vi "moving average.vi"(8 "error in (no error)":errorcluster, 10 "window size (3)":u32=3, 11 "x":dbl[](array[numeric])) -> (0 "error out":errorcluster, 3 "x smoothed":dbl[](array[numeric]))   [LabVIEW 2021]
uses:
  <vilib>/Analysis/2dsp.llb/1D Convolution (DBL).vi
  <vilib>/Analysis/NI_AALPro.lvlib
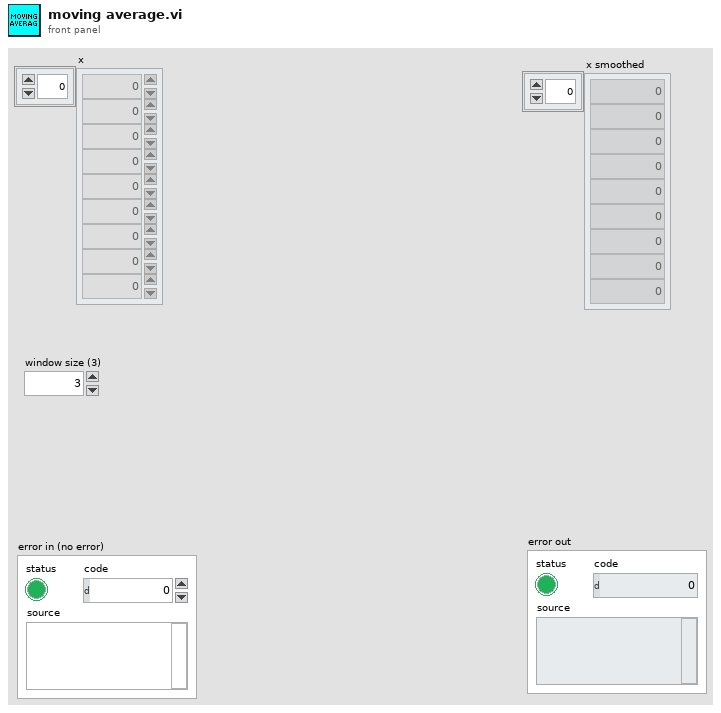
[diagram p1: front panel]
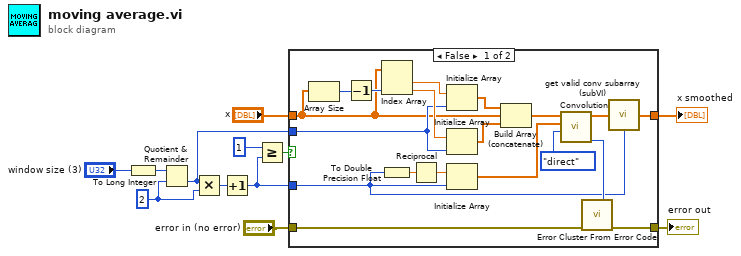
[diagram p0: block diagram]
diagram:
  w12 = 2 ("y")
  n1 = To Long Integer(number="window size (3)") -> (32bit integer=w10:i32)
  n2 = Quotient & Remainder(x=w10, y=w12) -> (floor(x/y)=w3:i32)  [unwired: 1 out]
  n3 = Multiply(x=w3, y=w12) -> (x*y=w2:i32)
  n4 = Increment(x=w2) -> (x+1=w8:i32)
  n5 = Greater Or Equal?(x=1, y=w8) -> (x >= y?=w7:bool)
  n6 = case shown="False" w7 {
    tunnel: w8 -> [w15 _]
    tunnel: [w14 w33] -> w5
    tunnel: "x" -> [w13 w33]
    tunnel: "error in (no error)" -> [w20 w32]
    tunnel: [w19 w32] -> w1
    tunnel: w3 -> [w16 _]
    frame False {
      n7 = Array Size(array=w13) -> (size(s)=w17:i32)
      n8 = Decrement(x=w17) -> (x-1=w28:i32)
      n9 = Index Array(array=w13, index #2=w28) -> (element #1=w29:dbl, element #2=w27:dbl)  [unwired: 1 in]
      n10 = To Double Precision Float(number=w15) -> (double precision float=w31:dbl)
      n11 = Reciprocal(x=w31) -> (1/x=w30:dbl)
      n12 = Initialize Array(w29, w16) -> (w26:dbl[])
      n13 = Initialize Array(w27, w16) -> (w25:dbl[])
      n14 = Initialize Array(w30, w15) -> (w24:dbl[])
      n15 = Build Array (concatenate)(w26, w13, w25) -> (w23:dbl[])
      n16 = call-poly <vilib>:"Convolution.vi"("algorithm"=enum32{"direct", "frequency domain"}."direct", "Y"=w24, "X"=w23) -> ("error"=w21:i32, "X * Y"=w18:dbl[])  [unwired: 7 in]
      n17 = call <vilib>:"Error Cluster From Error Code.vi"("error in (no error)"=w20, "error code (0)"=w21) -> ("error out"=w19:errorcluster)  [unwired: 7 in]
      n18 = call "get valid conv subarray (subVI).vi"("k size"=w15, "X * k"=w18) -> ("X * k valid"=w14:dbl[])  [unwired: 2 in]
    }
    frame True {
    }
  }
  "x smoothed" <- w5
  "error out" <- w1
